vi "dice.vi"(2 "PUSH Button":bool) -> (1 "Dice":dbl)   [LabVIEW 2014]
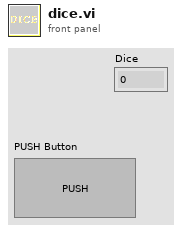
[diagram p1: front panel]
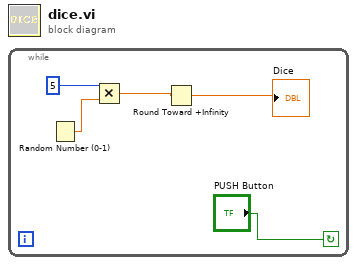
[diagram p0: block diagram]
diagram:
  n1 = while {
    stop <- "PUSH Button" continue-if-true
    n2 = Random Number (0-1)() -> (number: 0 to 1=w4:dbl)
    n3 = Multiply(x=5, y=w4) -> (x*y=w3:dbl)
    n4 = Round Toward +Infinity(x=w3) -> (ceil(x): smallest int >= x=→"Dice":dbl)
  }
